vi "NI 5783 - Getting Started (Host).vi"() -> ()   [LabVIEW 2017]
uses:
  <vilib>/userdefined/Silver/nirio_resource_slv.ctl
  Program Files (x86)/National Instruments/LabVIEW 2017/examples/FlexRIO/IO Modules/NI 5783/NI 5783 - Getting Started/Controls/Clock Select.ctl
  <vilib>/FPGAPlugInAG/PXIe-7976R/niLvFpga_Open_PXIe-7976R.vi
  <vilib>/rvi/interface/common/dynamic/niFpgaDynamicAddResources.vi
  <vilib>/rvi/interface/common/niFpgaWaitOnOcc.vi
  <vilib>/Utility/error.llb/Error Cluster From Error Code.vi
  <vilib>/rvi/errors/niLvFpgaAdjustHostInterfaceError.vi
  <instrlib>/_niInstr/Streaming/v1/Host/Public/Start Finite Stream.vi
  <instrlib>/_niInstr/Streaming/v1/Host/Public/Wait for Stream.vi
  <vilib>/FPGAPlugInAG/Dynamic/niLvFpga_Close_Dynamic.vi
  <vilib>/rvi/interface/nirviOpenFPGA/nirviOpenFPGA.xnode
  FPGA Bitfiles/ADCSamples_FPGATarget_NI5783-GettingSt_O3Cot-WQFrs.lvbitx
  <vilib>/rvi/interface/nirviMethod/nirviMethod.xnode
  <vilib>/rvi/interface/nirviReadWriteControl/nirviReadWriteControl.xnode
  <vilib>/rvi/interface/nirviCloseFPGA/nirviCloseFPGA.xnode
  <vilib>/rvi/errors/niLvFpgaMergeErrorWithErrorCode.vi
  <instrlib>/_niInstr/Streaming/v1/Host/niInstr Streaming v1 Host.lvlib
  <vilib>/FPGAPlugInAG/Dynamic/niLvFpga_ConfigureFifo_Dynamic.vi
  <vilib>/FPGAPlugInAG/Dynamic/niLvFpga_StartFifo_Dynamic.vi
  NiFpgaLv.dll
  <vilib>/rvi/interface/Simulation/niFpgaSimulationCallBeginRW.vi
  <vilib>/FPGAPlugInAG/Dynamic/niLvFpga_ReadFifo_Dynamic.vi
panel:
  out "Samples Acquired":i32=4096
  in  "Samples to Acquire":u64=4096
  in  "Trigger Type":enum8{"Immediate", "Data Trigger", "TRIG input"}(ring)
  in  "Clock Select":T1 items=["Internal Clock", "Internal Clock w/ Ref via CLK/REF IN", "Internal Clock w/ Ref via Sync Clock", "External Clock via CLK/REF IN"]
  in  "Rate of External Sample Clock (MHz)":u16=100 min=60 max=100 step=1
  in  "Data Trigger When":enum8{"Trigger Above", "Trigger Below"}(ring)
  out "AI":waveform(dbl)[](graph)
  out "Error Out":errorcluster
  in  "Data Trigger Level (V)":dbl
  in  "stop":bool
  in  "Record Size":u64=4096
  in  "RIO Resource":T2="RIO0"
  # "Resource Configuration"
  # "AI Configuration"
  # "Ignored when Internal Clock is selected"
  # "AI Configuration"
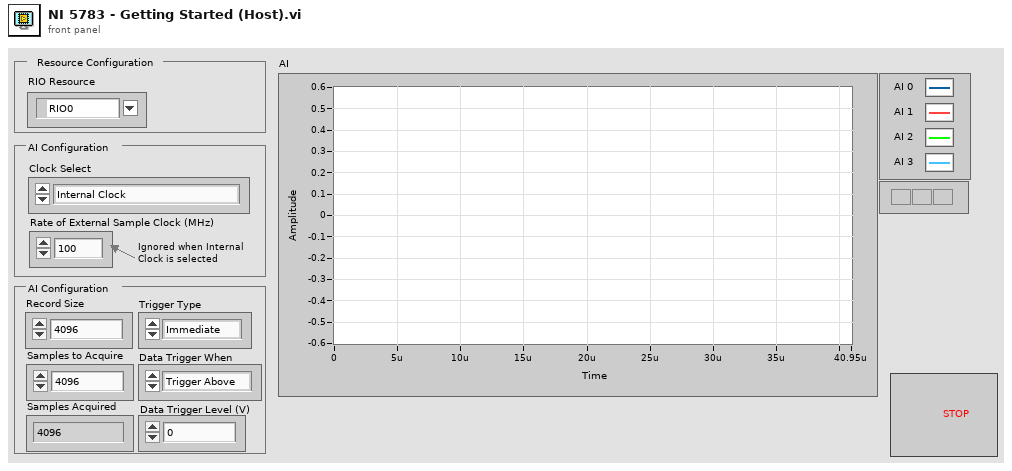
[diagram p1: front panel]
types:
  T1 = typedef "Clock Select.ctl" = u16
  T2 = typedef "nirio_resource_slv.ctl" = tag
  T3 = cluster{"level":i16, "trigger when":enum8{"Trigger Above", "Trigger Below"}}
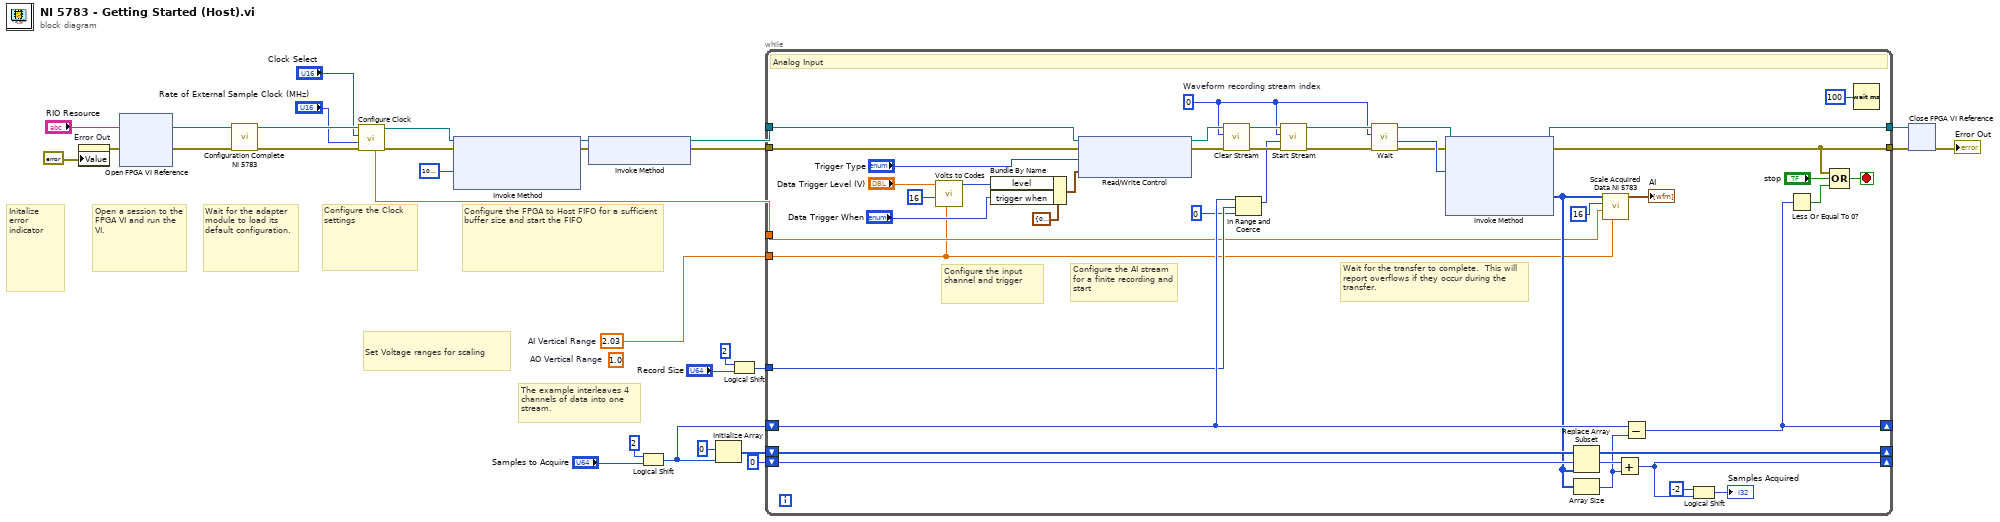
[diagram p0: block diagram]
diagram:
  w21 = 2.03  # AI Vertical Range
  (unwired) 1.0  # AO Vertical Range
  # "The example interleaves 4 channels of data into one stream."
  # "Configure the Clock settings"
  # "Configure the FPGA to Host FIFO for a sufficient buffer size and start the FIFO"
  # "Wait for the adapter module to load its default configuration."
  # "Open a session to the FPGA VI and run the VI."
  # "Set Voltage ranges for scaling"
  # "Initalize error indicator"
  n1 = property on="Error Out" class="Clust (strict)"("Value"=errorcluster {"status"=FALSE, "code"=0, "source"=""} ("error out")) -> (error out=w28:errorcluster)  [unwired: 2 in, 1 out]
  n2 = xnode "Open FPGA VI Reference"("error in"=w28, "resource name"="RIO Resource") -> ("FPGA VI Reference Out"=w20:refnum<k20>, "error out"=w19:errorcluster)
  n3 = call "Configuration Complete NI 5783.vi"("error in"=w19, "FPGA VI Reference In"=w20) -> ("error out"=w17:errorcluster, "FPGA VI Reference Out"=w18:refnum<k20>)  [unwired: 7 in, 1 out]
  n4 = call "Configure Clock.vi"("error in (no error)"=w17, "Rate of External Sample Clock (MHz)"="Rate of External Sample Clock (MHz)", "Clock Select"="Clock Select", "FPGA VI Reference In"=w18) -> ("error out"=w15:errorcluster, "FPGA VI Reference Out"=w16:refnum<k20>, "Sampling Rate"=w12:dbl)  [unwired: 3 in, 2 out]
  n5 = xnode "Invoke Method"("FPGA VI Reference In"=w16, "error in"=w15, "Requested Depth"=u32 1024000) -> ("FPGA VI Reference Out"=w24:refnum<k20>, "error out"=w23:errorcluster)  [unwired: 1 out]
  n6 = xnode "Invoke Method"("FPGA VI Reference In"=w24, "error in"=w23) -> ("FPGA VI Reference Out"=w26:refnum<k20>, "error out"=w25:errorcluster)
  n7 = Logical Shift(y=u16 2, x="Samples to Acquire") -> (x << y=w5:u64)
  n8 = Initialize Array(i16 0 ("element"), w5) -> (w9:i16[])
  n9 = Logical Shift(y=u16 2, x="Record Size") -> (x << y=w2:u64)
  n10 = while {
    tunnel: [w71] -> w30
    tunnel: w26 -> [w70]
    tunnel: w21 -> [w36]
    tunnel: w25 -> [w69]
    tunnel: [w58] -> w11
    tunnel: w12 -> [w37]
    shift-right: [w46] -> _
    shift-left: w5 -> [w41]
    shift-right: [w43] -> _
    shift-left: w9 -> [w44]
    shift-right: [w35] -> _
    shift-left: 0 ("index") -> [w42]
    tunnel: w2 -> [w40]
    stop <- w47 stop-if-true
    w48 = 0  # Waveform recording stream index
    # "Wait for the transfer to complete.  This will report overflows if they occur during the transfer."
    # "Configure the AI stream for a finite recording and start"
    # "Configure the input channel and trigger"
    # "Analog Input"
    n11 = call "Volts to Codes.vi"("range (Vpp)"=w36, "Number of Bits"=i16 16, "Volts In"="Data Trigger Level (V)") -> ("ADC Codes Out"=w54:i16)  [unwired: 8 in]
    n12 = Bundle By Name(cluster=T3 {"level"=0, "trigger when"=enum."Trigger Above"} ("Trigger Configuration"), "level"=w54, "trigger when"="Data Trigger When") -> (w57:T3)
    n13 = xnode "Read/Write Control"("FPGA VI Reference In"=w70, "error in"=w69, "Trigger Type"="Trigger Type", "Trigger Configuration"=w57) -> ("FPGA VI Reference Out"=w52:refnum<k20>, "error out"=w51:errorcluster)
    n14 = call <instrlib>:"Clear Stream.vi"("error in (no error)"=w51, "stream index"=w48, "refnum in"=w52) -> ("error out"=w50:errorcluster, "refnum out"=w49:refnum<k20>)  [unwired: 7 in]
    n15 = In Range and Coerce(upper limit=w41, x=w40, lower limit=u64 0) -> (coerced(x)=w31:u64)  [unwired: 1 out]
    n16 = call-poly <instrlib>:"Start Stream.vi"("error in (no error)"=w50, "num samples"=w31, "stream index"=w48, "refnum in"=w49) -> ("error out"=w63:errorcluster, "refnum out"=w61:refnum<k20>)  [unwired: 6 in]
    n17 = call-poly <instrlib>:"Wait.vi"("error in (no error)"=w63, "stream index"=w48, "refnum in"=w61) -> ("error out"=w59:errorcluster, "samples transferred"=w62:u64, "refnum out"=w60:refnum<k20>)  [unwired: 5 in, 1 out]
    n18 = xnode "Invoke Method"("FPGA VI Reference In"=w60, "error in"=w59, "Number of Elements"=w62) -> ("FPGA VI Reference Out"=w71:refnum<k20>, "error out"=w58:errorcluster, "Data"=w38:i16[])  [unwired: 1 in, 1 out]
    n19 = Replace Array Subset(array=w44, new element=w38, index=w42) -> (w43:i16[])
    n20 = Array Size(array=w38) -> (size(s)=w39:i32)
    n21 = call "Scale Acquired Data NI 5783.vi"("range (V)"=w36, "Sample Rate"=w37, "Number of Bits"=i16 16, "Data In"=w38) -> ("Data"=→"AI":waveform(dbl)[])  [unwired: 7 in]
    n22 = Add(x=w42, y=w39) -> (x+y=w35:i32)
    n23 = Subtract(x=w41, y=w39) -> (x-y=w46:u64)
    n24 = Logical Shift(y=i16 -2, x=w35) -> (x << y=→"Samples Acquired":i32)
    n25 = Less Or Equal To 0?(x=w46) -> (x <= 0?=w45:bool)
    n26 = Compound Arithmetic op=OR(w58, "stop", w45) -> (w47:bool)
    n27 = Wait (ms)(milliseconds to wait=u32 100) -> ()  [unwired: 1 out]
  }
  n28 = xnode "Close FPGA VI Reference"("FPGA VI Reference In"=w30, "error in"=w11) -> ("error out"=→"Error Out":errorcluster)
